vi "To String.vi"(8 "error in (no error)":errorcluster, 11 "Cluster in":refnum<class "Cluster.lvclass">) -> (0 "error out":errorcluster, 2 "String":string)   [LabVIEW 2020, in "Data.lvlib" / "Cluster.lvclass"]
doc: "Convert 'Generic Data in' to a string.\nThe default implementation convert the data to an XML string."
uses:
  Cluster.lvclass
  Cluster.lvclass/Cluster.ctl
  Generic Data.lvclass
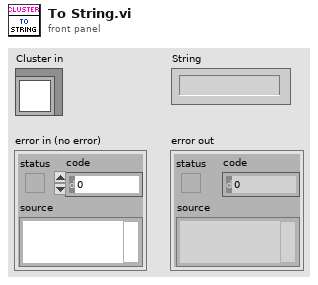
[diagram p1: front panel]
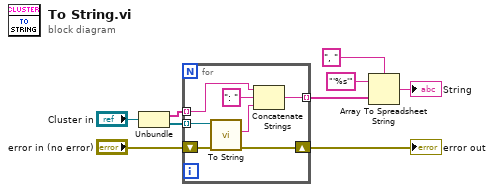
[diagram p0: block diagram]
diagram:
  n1 = Unbundle("Cluster in") -> (w7:string[], w8:refnum<class "Generic Data.lvclass">[])
  n2 = for {
    tunnel: w8 -> [w16] mode=indexing
    tunnel: w7 -> [w15] mode=indexing
    shift-right: [w11] -> w5
    shift-left: "error in (no error)" -> [w12]
    tunnel: [w10] -> w2 mode=indexing
    n3 = call-dynamic "To String.vi"("error in (no error)"=w12, "Generic Data in"=w16) -> ("error out"=w11:errorcluster, "String"=w13:string)  [unwired: 8 in]
    n4 = Concatenate Strings(w15, ": " ("string"), w13) -> (w10:string)
  }
  "error out" <- w5
  n5 = Array To Spreadsheet String(delimiter (Tab)=", ", array=w2, 3:"'%s'" ("format string")) -> (spreadsheet string=→"String":string)
